vi "NFILE2.vi"() -> ()   [LabVIEW 2019]
uses:
  Control 3.ctl
  Control 1.ctl
panel:
  out "Fáze":dbl
  in  "Fvz":T1=1000.0
  in  "Sirka okna (ms)":i32(listbox)
  in  "Offset":dbl format="%0.2p"
  in  "Amplituda sumu":T2
  in  "Amplituda":dbl=1.0 format="%0.2p"
  in  "Frekvence":dbl=10.0 format="%0.2p"
  out "Waveform Graph 2":waveform(dbl)(graph)
  out "Waveform Graph":waveform(dbl)(graph)
  out "dt":dbl
  out "Boolean":bool=TRUE
  out "remaining elements":dbl[](array[numeric])
  in  "stop":bool
  out "# elements in queue":i32
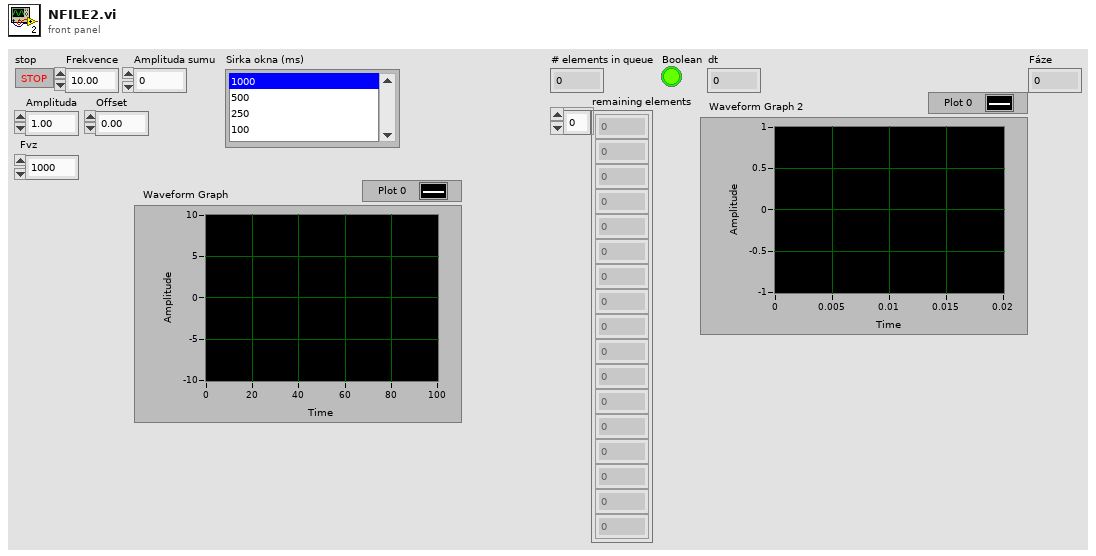
[diagram p1: front panel]
types:
  T1 = typedef "Control 1.ctl" = dbl
  T2 = typedef "Control 3.ctl" = dbl
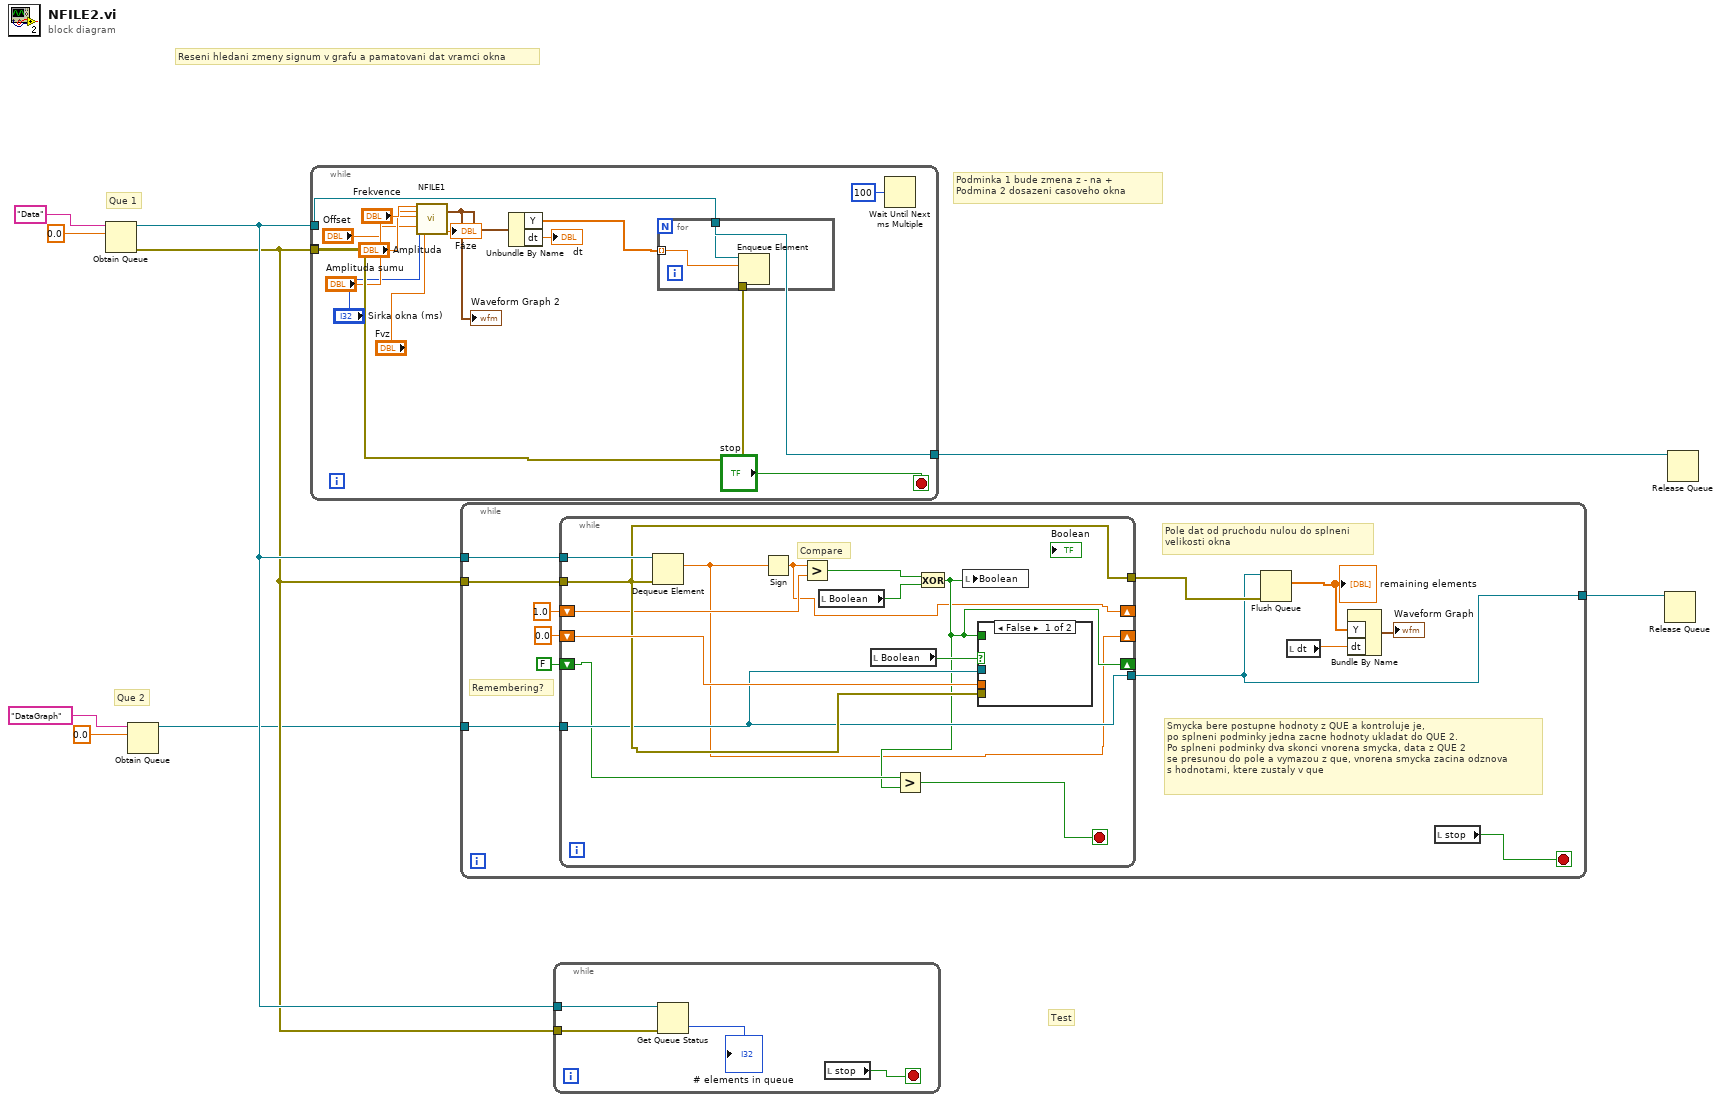
[diagram p0: block diagram]
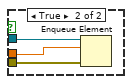
[diagram p2: hidden frame]
diagram:
  # "Test"
  # "Podminka 1 bude zmena z - na +\nPodmina 2 dosazeni casoveho okna"
  # "Reseni hledani zmeny signum v grafu a pamatovani dat vramci okna"
  # "Que 1"
  # "Que 2"
  n1 = Obtain Queue(name (unnamed)="Data", element data type=0.0) -> (queue out=w7:refnum<queue>, error out=w6:errorcluster)  [unwired: 3 in, 1 out]
  n2 = Obtain Queue(name (unnamed)="DataGraph", element data type=0.0) -> (queue out=w3:refnum<queue>)  [unwired: 3 in, 2 out]
  n3 = while {
    tunnel: w7 -> [w22]
    tunnel: [w23] -> _
    tunnel: w6 -> [w23]
    tunnel: [w22] -> w1
    stop <- "stop" stop-if-true
    n4 = call "NFILE1.vi"("Frekvence"="Frekvence", "Amplituda"="Amplituda", "Amplituda sumu"="Amplituda sumu", "Offset"="Offset", "Sirka okna (ms)"="Sirka okna (ms)", "Fvz"="Fvz") -> ("Fáze"=→"Fáze":dbl, "Waveform Graph"=w17:waveform(dbl))  [unwired: 12 in]
    "Waveform Graph 2" <- w17
    n5 = Unbundle By Name(w17) -> ("Y"=w19:dbl[], "dt"=→"dt":dbl)
    n6 = for {
      tunnel: w23 -> [w26]
      tunnel: w22 -> [w25]
      tunnel: w19 -> [w24] mode=indexing
      n7 = Enqueue Element(queue=w25, element=w24, error in (no error)=w26) -> ()  [unwired: 1 in, 3 out]
    }
    n8 = Wait Until Next ms Multiple(millisecond multiple=u32 100) -> ()  [unwired: 1 out]
  }
  n9 = while {
    tunnel: w7 -> [w38]
    tunnel: w6 -> [w37]
    tunnel: w3 -> [w34]
    tunnel: [w32] -> w2
    stop <- w31 stop-if-true
    # "Pole dat od pruchodu nulou do splneni\nvelikosti okna"
    # "Smycka bere postupne hodnoty z QUE a kontroluje je,\npo splneni podminky jedna zacne hodnoty ukladat do QUE 2.\nPo splneni podminky dva skonci vnorena smycka, data z QUE 2 \nse presunou do pole a vymazou z que, vnorena smycka zacina odznova\ns hodnotami, ktere zustaly v que"
    # "Remembering?"
    n10 = while {
      tunnel: w38 -> [w51]
      tunnel: w37 -> [w49]
      shift-right: [w40] -> _
      shift-left: 0.0 -> [w50]
      shift-right: [w42] -> _
      shift-left: FALSE -> [w43]
      tunnel: w34 -> [w48]
      tunnel: [w49] -> w33
      tunnel: [w48] -> w32
      shift-right: [w39] -> _
      shift-left: 1.0 -> [w47]
      stop <- w41 stop-if-true
      # "Compare"
      n11 = Dequeue Element(queue=w51, error in (no error)=w49) -> (element=w40:dbl)  [unwired: 1 in, 3 out]
      n12 = Sign(1:w40) -> (0:w39:dbl)
      n13 = Greater?(x=w39, y=w47) -> (0:w46:bool)
      n14 = local read "Boolean"() -> (w45:bool)
      n15 = local read "Boolean"() -> (w44:bool)
      n16 = Exclusive Or(1:w45, 2:w46) -> (0:w42:bool)
      n17 = Greater?(x=w43, y=w42) -> (0:w41:bool)
      n18 = local write "Boolean"(w42) -> ()
      n19 = case shown="False" w44 {
        tunnel: w50 -> [_ w53]
        tunnel: w48 -> [_ w54]
        tunnel: w49 -> [_ w52]
        tunnel: w42 -> [_ _]
        frame False {
        }
        frame True {
          n20 = Enqueue Element(queue=w54, element=w53, error in (no error)=w52) -> ()  [unwired: 1 in, 3 out]
        }
      }
    }
    n21 = Flush Queue(queue=w32, error in (no error)=w33) -> (remaining elements=w28:dbl[])  [unwired: 2 out]
    "remaining elements" <- w28
    n22 = local read "dt"() -> (w29:dbl)
    n23 = Bundle By Name("Y"=w28, "dt"=w29) -> (→"Waveform Graph":waveform(dbl))  [unwired: 1 in]
    n24 = local read "stop"() -> (w31:bool)
  }
  n25 = while {
    tunnel: w7 -> [w58]
    tunnel: w6 -> [w57]
    stop <- w55 stop-if-true
    n26 = Get Queue Status(queue=w58, error in (no error)=w57) -> (# elements in queue=→"# elements in queue":i32)  [unwired: 1 in, 7 out]
    n27 = local read "stop"() -> (w55:bool)
  }
  n28 = Release Queue(queue=w2) -> ()  [unwired: 2 in, 3 out]
  n29 = Release Queue(queue=w1) -> ()  [unwired: 2 in, 3 out]
